vi "Sub Calculation.vi"(10 "On/Off":bool, 11 "Numeric in":dbl) -> (2 "String":string, 3 "Numeric out":dbl)   [LabVIEW 2017]
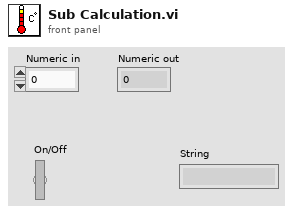
[diagram p1: front panel]
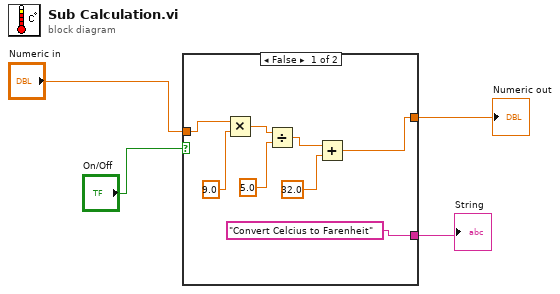
[diagram p0: block diagram]
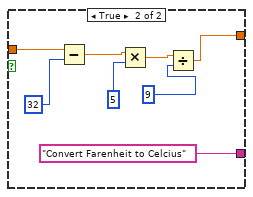
[diagram p2: hidden frame]
diagram:
  n1 = case shown="False" "On/Off" {
    tunnel: [w5 w20] -> w4
    tunnel: "Numeric in" -> [w9 w14]
    tunnel: ["Convert Celcius to Farenheit" "Convert Farenheit to Celcius"] -> w1
    frame False {
      n2 = Multiply(x=w9, y=9.0) -> (x*y=w8:dbl)
      n3 = Divide(x=w8, y=5.0) -> (x/y=w7:dbl)
      n4 = Add(x=w7, y=32.0) -> (x+y=w5:dbl)
    }
    frame True {
      n5 = Subtract(x=w14, y=32) -> (x-y=w18:dbl)
      n6 = Multiply(x=w18, y=5) -> (x*y=w19:dbl)
      n7 = Divide(x=w19, y=9) -> (x/y=w20:dbl)
    }
  }
  "Numeric out" <- w4
  "String" <- w1
